vi "ReadXLS_LogFiles.vi"() -> ()   [LabVIEW 2015, in "RW_Protocols.lvlib"]
uses:
  RW_Protocols.lvlib
  <vilib>/Utility/file.llb/Read Delimited Spreadsheet (DBL).vi
panel:
  out "all rows":dbl[][](array[numeric])
  out "Full File Path":path
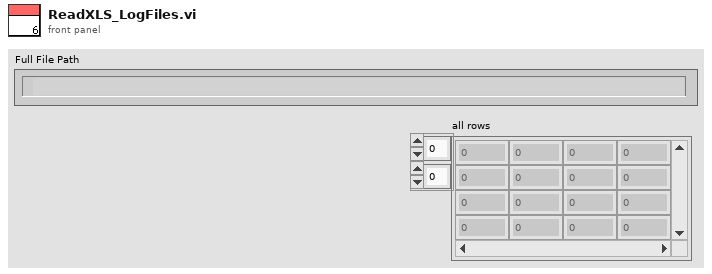
[diagram p1: front panel]
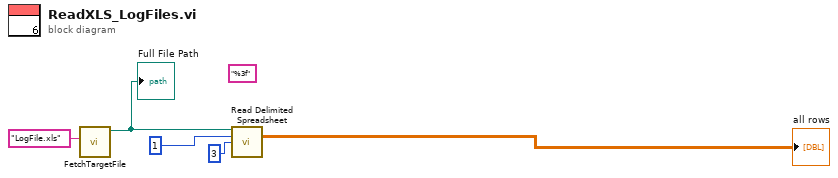
[diagram p0: block diagram]
diagram:
  (unwired) "%3f" ("format (%s)")
  n1 = call "FetchTargetFile.vi"("FileName"="LogFile.xls") -> ("Full File Path"=w4:path)  [unwired: 10 in]
  "Full File Path" <- w4
  n2 = call-poly <vilib>:"Read Delimited Spreadsheet.vi"("file path (dialog if empty)"=w4, "number of rows (all:-1)"=1, "start of read offset (chars.:0)"=3) -> ("all rows"=→"all rows":dbl[][])  [unwired: 7 in, 5 out]
